vi "getVelocityThresholds.vi"(8 "error in":errorcluster, 11 "connection ID":refnum<k5>) -> (0 "error out":errorcluster, 1 "velocityOff":i32, 2 "velocityOn":i32, 3 "connection ID":refnum<k5>)   [LabVIEW 2016]
doc: "Returns the threshold velocity (in µm/s) for mode 2 of setDynamicNormalization."
panel:
  out "params_cluster":cluster{"Numeric":i32}
  in  "Params_cluster":cluster{"Numeric":dbl}
  in  "results_cluster":T1
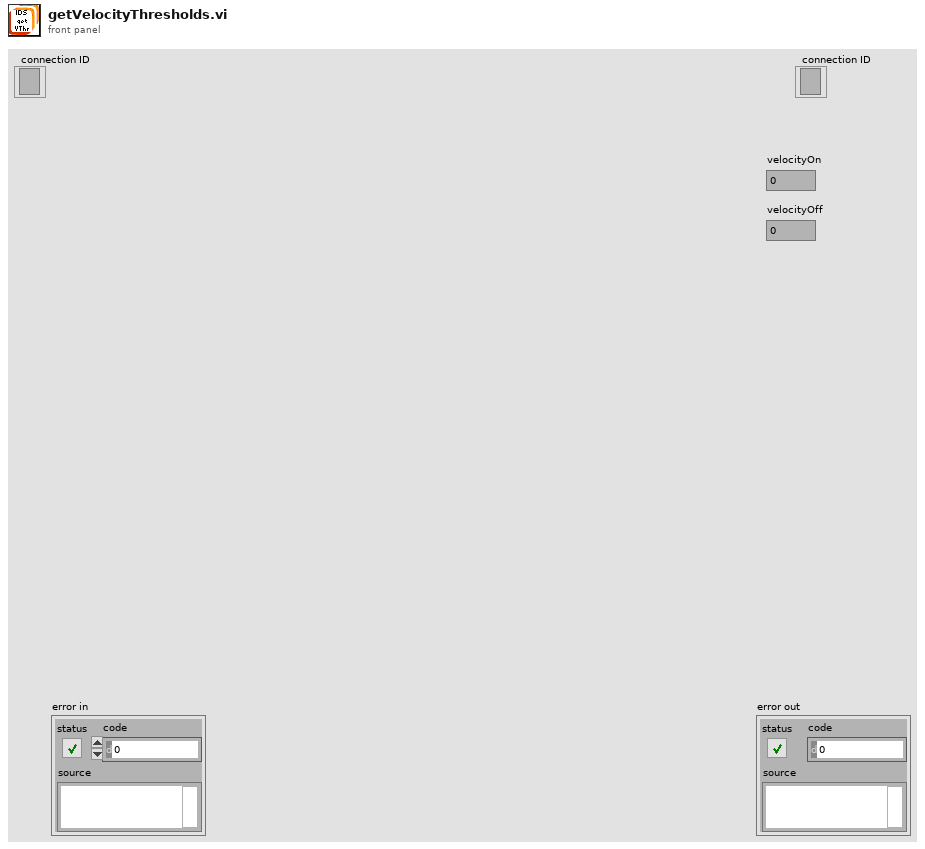
[diagram p1: front panel]
types:
  T1 = cluster{"errNo":i32, "velocityOn":i32, "velocityOff":i32}
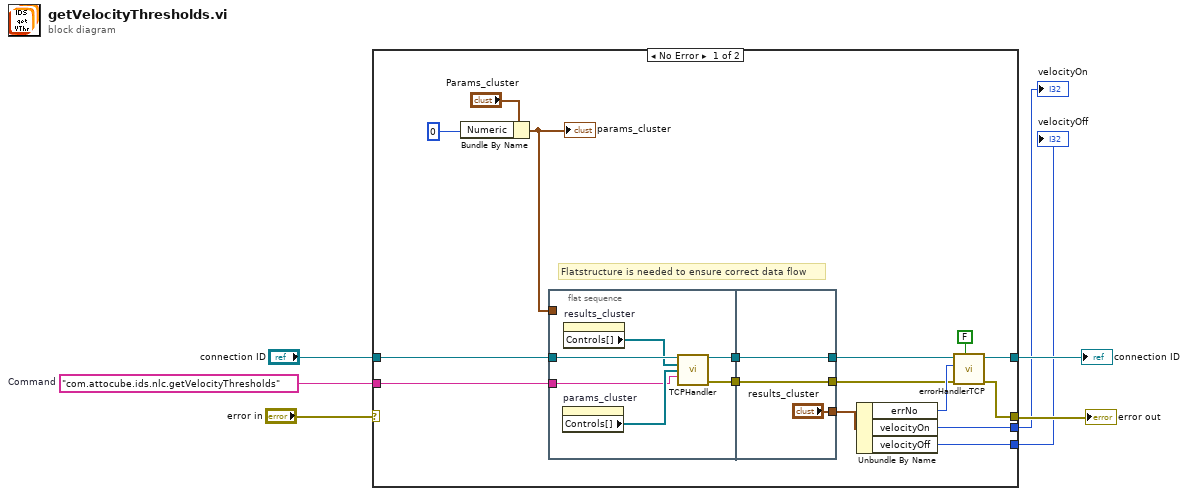
[diagram p0: block diagram]
diagram:
  w3 = "com.attocube.ids.nlc.getVelocityThresholds"  # Command
  n1 = case shown="No Error" "error in" {
    selector: "error in" -> [_ w34]
    tunnel: [w21 w34] -> w7
    tunnel: [w23 w33] -> w6
    tunnel: "connection ID" -> [w20 w33]
    tunnel: w3 -> [w14 _]
    tunnel: [w9 _] -> w2
    tunnel: [w8 _] -> w1
    frame No Error {
      # "Flatstructure is needed to ensure correct data flow"
      n2 = Bundle By Name(cluster="Params_cluster", "Numeric"=0) -> (w11:cluster{"Numeric":dbl})
      "params_cluster" <- w11
      n3 = flat-sequence {
        tunnel: [w28] -> w16
        tunnel: w20 -> [w29]
        tunnel: w14 -> [w25]
        tunnel: [w24] -> w12
        tunnel: w11 -> [_]
        tunnel: ["results_cluster"] -> w17
        tunnel: [w32] -> w19
        tunnel: w16 -> [w32]
        tunnel: [w30] -> w13
        tunnel: w12 -> [w30]
        frame #0 {
          n4 = property on="params_cluster" class="Clust (strict)"() -> ("Controls[]"=w26:refnum<vi>[])  [unwired: 2 in, 2 out]
          n5 = property on="results_cluster" class="Clust (strict)"() -> ("Controls[]"=w27:refnum<vi>[])  [unwired: 2 in, 2 out]
          n6 = call "TCPHandler.vi"("connection ID"=w29, "results_cluster"=w27, "params_cluster"=w26, "method"=w25) -> ("connection ID"=w28:refnum<k5>, "error"=w24:errorcluster)  [unwired: 8 in, 2 out]
        }
        frame #1 {
        }
      }
      n7 = Unbundle By Name(w17) -> ("errNo"=w18:i32, "velocityOn"=w9:i32, "velocityOff"=w8:i32)
      n8 = call "errorHandlerTCP.vi"("show popup"=FALSE, "error in"=w13, "error number"=w18, "connection ID"=w19) -> ("error out"=w21:errorcluster, "connection ID"=w23:refnum<k5>)  [unwired: 6 in]
    }
    frame Error {
    }
  }
  "error out" <- w7
  "connection ID" <- w6
  "velocityOn" <- w2
  "velocityOff" <- w1
